vi "Tell Parent.vi"(6 "Error":errorcluster, 7 "Actor Layer":refnum<class "Actor Layer.lvclass">, 9 "Payload":T10, 10 "Priority":bool, 11 "Actor":T1) -> (3 "Actor":T1, 4 "Error":errorcluster, 5 "Actor Layer":refnum<class "Actor Layer.lvclass">)   [LabVIEW 2020, in "_Template.lvlib" / "{{Msg}}.lvlib"]
uses:
  {{Msg}}.lvlib
  jettl/jettl/Msg/Msg.lvclass
  jettl/jettl/Metadata/Metadata.lvclass
  jettl/jettl/Origin.ctl
  jettl/jettl/jettl.lvlib
  jettl/jettl/Actor Layer/Actor Layer.lvclass
  Payload.ctl
  jettl/jettl/Msg.ctl
  jettl/jettl/Post Setup.ctl
  jettl/jettl/Pre Setup.ctl
  jettl/jettl/Msg Set.ctl
  jettl/jettl/Lifecycle.ctl
  jettl/jettl/Actor Attribs.ctl
  jettl/jettl/Children.ctl
  jettl/jettl/Actor.ctl
  jettl/jettl/Msg Attribs.ctl
  jettl/jettl/Layer Type.ctl
  jettl/jettl/Layer Attribs.ctl
  jettl/jettl/Layer Map.ctl
  jettl/jettl/Implemented Map.ctl
panel:
  # "This front panel should not be manipulated."
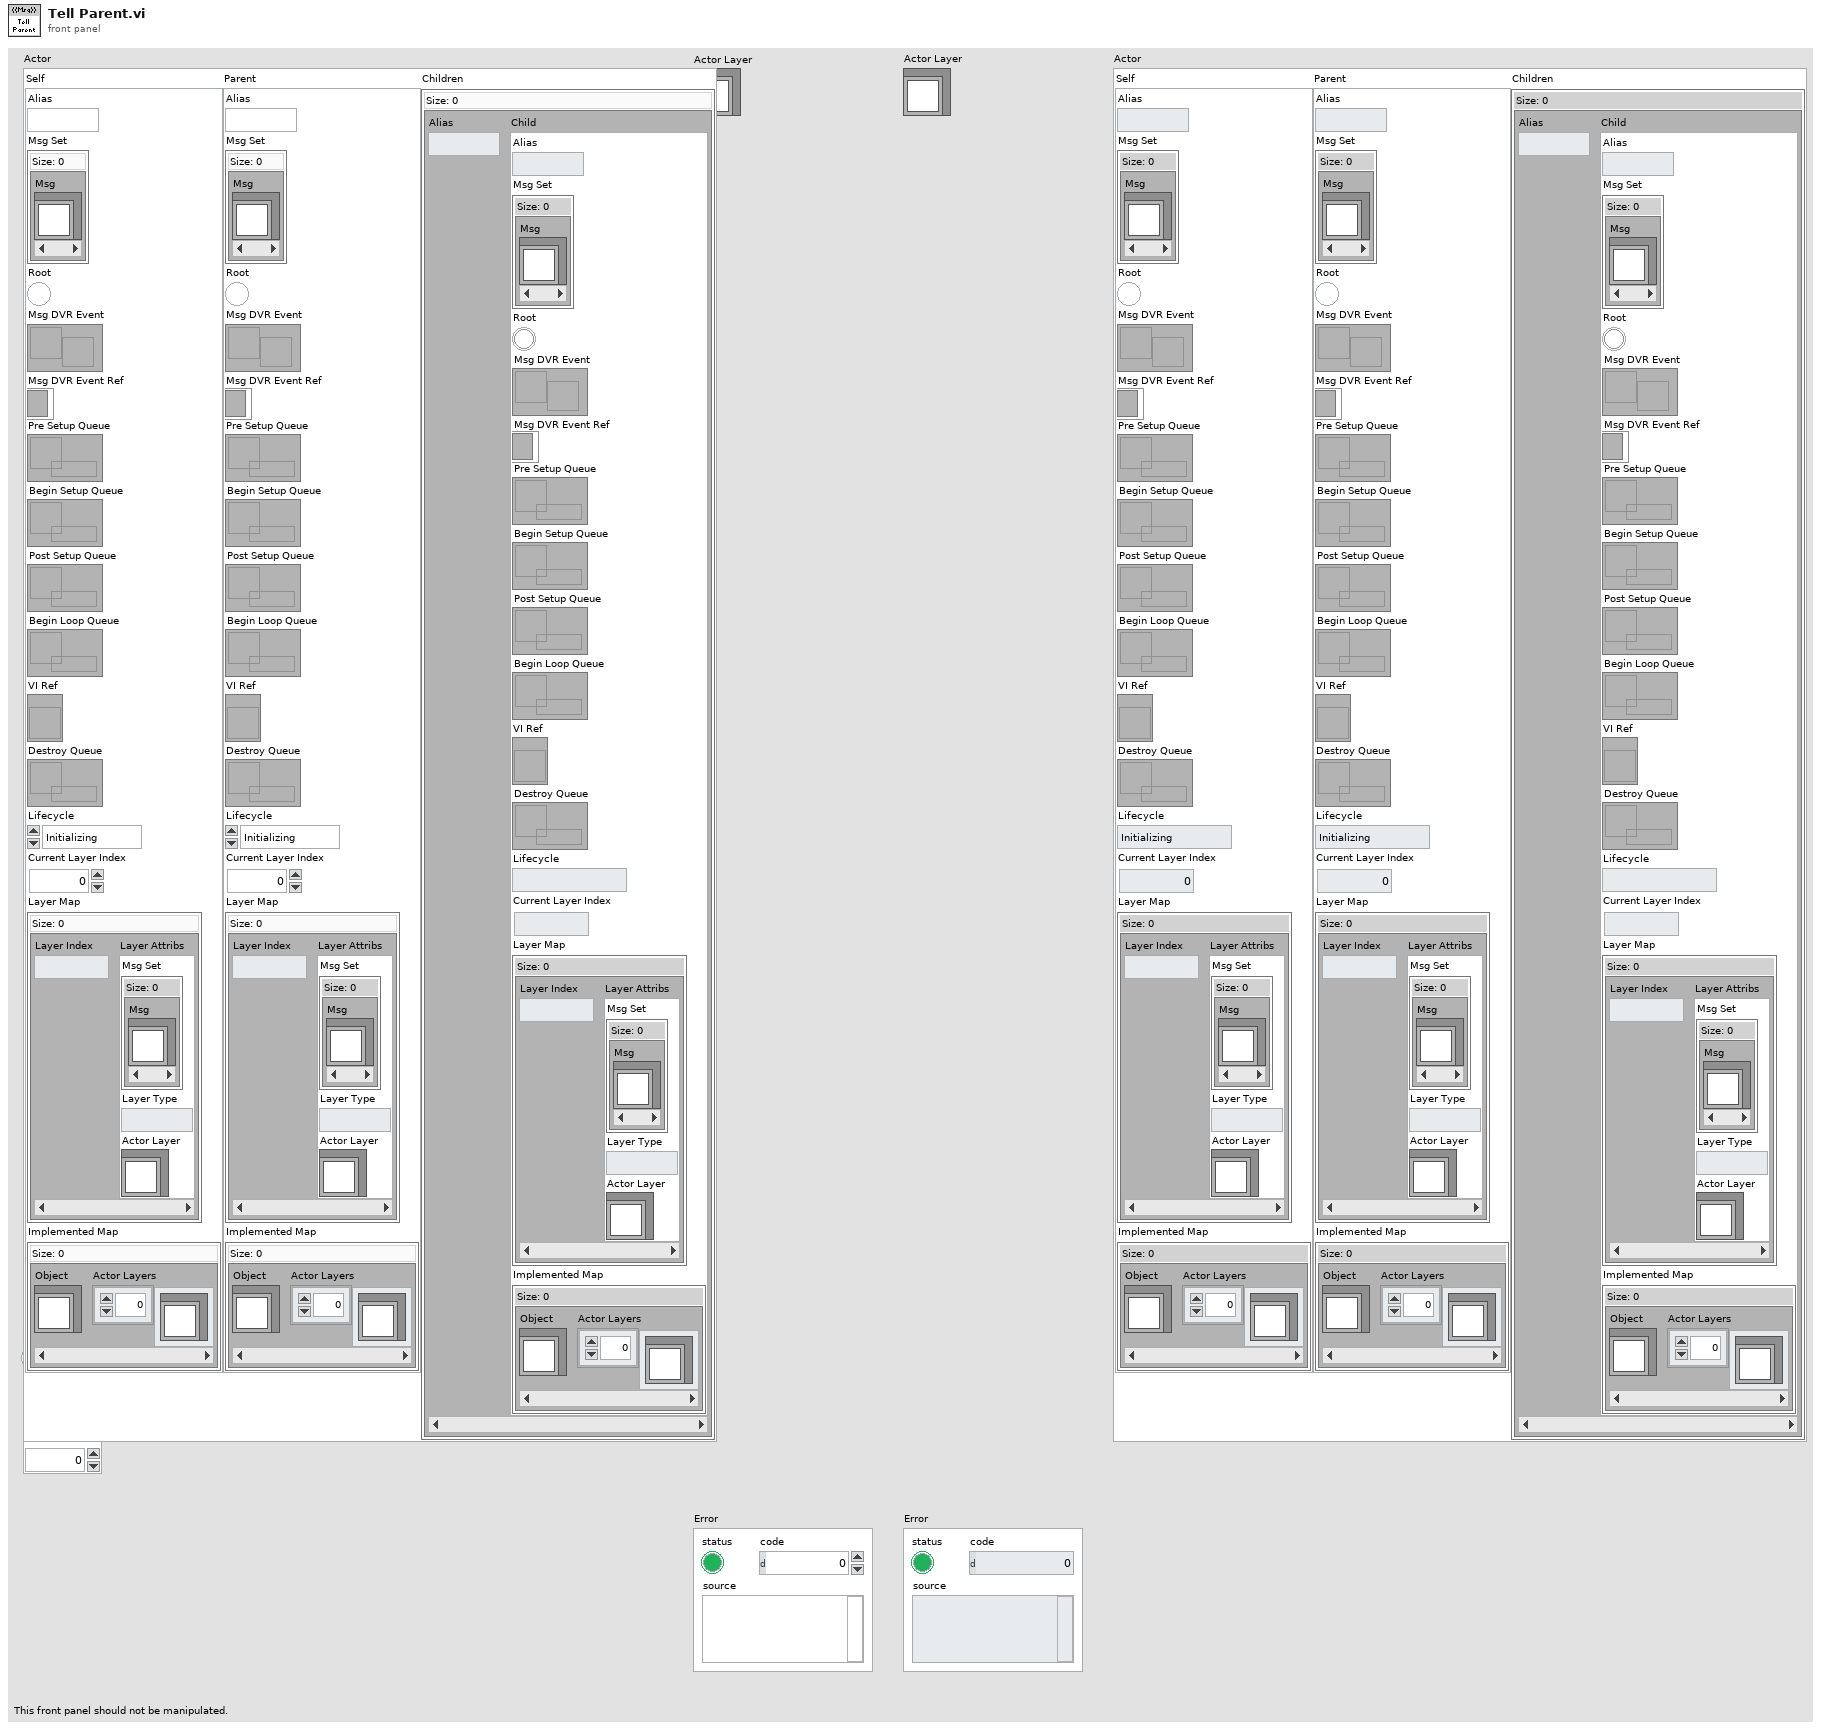
[diagram p1: front panel]
types:
  T1 = typedef "jettl.lvlib/Actor.ctl" = cluster{"Self":T2, "Parent":T2, "Children":T9}
  T2 = typedef "jettl.lvlib/Actor Attribs.ctl" = cluster{"Alias":string, "Msg Set":T3, "Root":bool, "Msg DVR Event":refnum<user-event>, "Msg DVR Event Ref":refnum<event-registration>, "Pre Setup Queue":refnum<queue>, "Begin Setup Queue":refnum<queue>, "Post Setup Queue":refnum<queue>, "Begin Loop Queue":refnum<queue>, "VI Ref":refnum<vi>, "Destroy Queue":refnum<queue>, "Lifecycle":T4, "Current Layer Index":i32, "Layer Map":T5, "Implemented Map":T8}
  T3 = typedef "jettl.lvlib/Msg Set.ctl" = set{refnum<class "Msg.lvclass">}
  T4 = typedef "jettl.lvlib/Lifecycle.ctl" = enum16{"Initializing", "Setting Up", "Starting", "Running", "Stopping", "Tearing Down", "Terminated"}
  T5 = typedef "jettl.lvlib/Layer Map.ctl" = map{i32, T6}
  T6 = typedef "jettl.lvlib/Layer Attribs.ctl" = cluster{"Msg Set":T3, "Layer Type":T7, "Actor Layer":refnum<class "Actor Layer.lvclass">}
  T7 = typedef "jettl.lvlib/Layer Type.ctl" = enum16{"Base", "InnerGlobal", "InnerLocal", "Outer"}
  T8 = typedef "jettl.lvlib/Implemented Map.ctl" = map{refnum<class>, refnum<class "Actor Layer.lvclass">[]}
  T9 = typedef "jettl.lvlib/Children.ctl" = map{string, T2}
  T10 = typedef "_Template.lvlib/{{Msg}}.lvlib/Payload.ctl" = cluster{"{{-}}":u8}
  T11 = typedef "jettl.lvlib/Origin.ctl" = enum16{"Self", "Parent", "Child"}
  T12 = typedef "jettl.lvlib/Msg.ctl" = cluster{"Msg Attribs DVR":refnum<data-value>, "Msg Attribs":T13, "Msg":refnum<class "Msg.lvclass">, "Msg Default":refnum<class "Msg.lvclass">}
  T13 = typedef "jettl.lvlib/Msg Attribs.ctl" = cluster{"Priority":bool, "Listener Alias":string, "Teller Alias":string, "Teller Lifecycle":T4, "Teller Origin":T11, "Tell Absolute Time":timestamp, "Tell Relative Time":dbl, "Listen Absolute Time":timestamp, "Listen Relative Time":dbl}
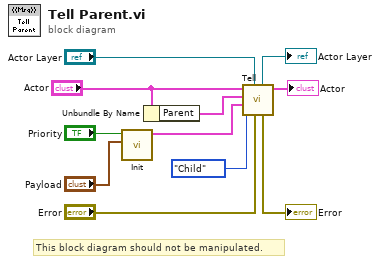
[diagram p0: block diagram]
diagram:
  # "This block diagram should not be manipulated."
  n1 = call "Init.vi"("Payload"="Payload", "Priority"="Priority") -> ("Msg"=w4:T12)  [unwired: 9 in]
  n2 = Unbundle By Name("Actor") -> ("Parent"=w10:T2)
  n3 = call "Tell.vi"("Error"="Error", "Actor Layer"="Actor Layer", "Origin"=Origin."Child" ("TellOrigin"), "Msg"=w4, "Actor Attribs"=w10, "Actor"="Actor") -> ("Actor"=→"Actor":T1, "Error"=→"Error":errorcluster, "Actor Layer"=→"Actor Layer":refnum<class "Actor Layer.lvclass">)  [unwired: 3 in]
